vi "final gps synchronization with recursive algorithm.vi"() -> ()   [LabVIEW 2014]
uses:
  <vilib>/FPGAPlugInAG/cRIO-9063/niLvFpga_Open_cRIO-9063.vi
  <vilib>/rvi/interface/common/dynamic/niFpgaDynamicAddResources.vi
  <vilib>/Utility/error.llb/Error Cluster From Error Code.vi
  <vilib>/rvi/errors/niLvFpgaAdjustHostInterfaceError.vi
  <vilib>/FPGAPlugInAG/Dynamic/niLvFpga_Close_Dynamic.vi
  <vilib>/rvi/interface/nirviOpenFPGA/nirviOpenFPGA.xnode
  akhil3/FPGA Bitfiles/trailswithgps_FPGATarget_recursiveakhil_QexfQQGvF84.lvbitx
  recursive akhil.vi
  akhil3/FPGA Bitfiles/trailswithgps_FPGATarget2_recursive2_3NDbUzkOS+M.lvbitx
  recursive2.vi
  <vilib>/rvi/interface/nirviReadWriteControl/nirviReadWriteControl.xnode
  <vilib>/rvi/interface/nirviCloseFPGA/nirviCloseFPGA.xnode
  NiFpgaLv.dll
  <vilib>/rvi/interface/Simulation/niFpgaSimulationCallBeginRW.vi
panel:
  out "Apparent Power":dynamicdata(graph)
  out "LabVIEW time":timestamp
  out "GPS status":T1(ring)
  out "FPGA Timekeeper locked":bool
  out "offset from time reference":i32
  out "Satellites Available":u8
  out "UTC offset":i8
  out "UTC offset valid":bool
  out "Frequency":fxp<+/-,35,18>
  out "current frequency":fxp<+/-,35,18>
  out "PPS Timestamp (TAI ns)":u64
  out "PPS TAI Timestamp":timestamp format="%<%.9X\n%x>T"
  out "PPS UTC Timestamp":timestamp format="%<%.9X\n%x>T"
  out "antenna status":T2(ring)
  out "Latitude (°)":fxp<+/-,28,8>
  out "Longitude (°)":fxp<+/-,29,9>
  out "Altitude (m)":fxp<+/-,24,17>
  out "ROCOF":fxp<+/-,17,17>
  out "Theta":fxp<+/-,22,10>[](array[numeric])
  out "Magnitude":fxp<+,60,17>[](array[numeric])
  out "Current Phasors":picture
  in  "polar attributes 6":T3={"maximum"=0.0, "minimum"=0.0, "clip to min"=FALSE, "log?(F)"=FALSE, "grid color"=6710886, "plot color"=65280, "fmt and prec"={"format"=enum."Decimal", "precision"=0}, "visible section"=8} {"minimum" format="%0.2f"; "maximum" format="%0.2f"}
  out "Voltage Phasors":picture
  in  "polar attributes 7":T3={"maximum"=0.0, "minimum"=0.0, "clip to min"=FALSE, "log?(F)"=FALSE, "grid color"=6710886, "plot color"=65280, "fmt and prec"={"format"=enum."Decimal", "precision"=0}, "visible section"=8} {"minimum" format="%0.2f"; "maximum" format="%0.2f"}
  out "?":cluster{fxp<+/-,22,10>[]}[](array[cluster])
  out "?":cluster{fxp<+,60,17>[]}[](array[cluster])
  out "?":cluster{fxp<+/-,22,10>[]}[](array[cluster])
  out "?":cluster{fxp<+,60,17>[]}[](array[cluster])
  out "Voltages at PMU 1":dynamicdata(graph)
  out "LabVIEW time 2":timestamp
  out "GPS status 2":T1(ring)
  out "FPGA Timekeeper locked 2":bool
  out "offset from time reference 2":i32
  out "Satellites Available 2":u8
  out "UTC offset 2":i8
  out "UTC offset valid 2":bool
  out "Frequency":fxp<+/-,35,18>
  out "current frequency 2":fxp<+/-,35,18>
  out "PPS Timestamp (TAI ns) 2":u64
  out "PPS TAI Timestamp 2":timestamp format="%<%.9X\n%x>T"
  out "PPS UTC Timestamp 2":timestamp format="%<%.9X\n%x>T"
  out "antenna status 2":T2(ring)
  out "Latitude (°) 2":fxp<+/-,28,8>
  out "Longitude (°) 2":fxp<+/-,29,9>
  out "Altitude (m) 2":fxp<+/-,24,17>
  out "ROCOF":fxp<+/-,17,17>
  out "Theta 2":fxp<+/-,22,10>[](array[numeric])
  out "Magnitude 2":fxp<+,60,17>[](array[numeric])
  out "Current Phasors":picture
  in  "polar attributes 8":T3={"maximum"=0.0, "minimum"=0.0, "clip to min"=FALSE, "log?(F)"=FALSE, "grid color"=6710886, "plot color"=65280, "fmt and prec"={"format"=enum."Decimal", "precision"=0}, "visible section"=8} {"minimum" format="%0.2f"; "maximum" format="%0.2f"}
  out "Voltage Phasors":picture
  in  "polar attributes 9":T3={"maximum"=0.0, "minimum"=0.0, "clip to min"=FALSE, "log?(F)"=FALSE, "grid color"=6710886, "plot color"=65280, "fmt and prec"={"format"=enum."Decimal", "precision"=0}, "visible section"=8} {"minimum" format="%0.2f"; "maximum" format="%0.2f"}
  out "?":cluster{fxp<+/-,22,10>[]}[](array[cluster])
  out "?":cluster{fxp<+,60,17>[]}[](array[cluster])
  out "?":cluster{fxp<+/-,22,10>[]}[](array[cluster])
  out "?":cluster{fxp<+,60,17>[]}[](array[cluster])
  out "Voltages at PMU 2":dynamicdata(graph)
  out "Frequency":dynamicdata(graph)
  out "Reactive Power":dbl
  out "Real Power":dbl
  out "Power factor":dbl
  out "Apparent Power":dbl
  out "Reactive Power":dbl
  out "Real Power":dbl
  out "Power factor":dbl
  out "Apparent Power":dbl
  out "Load angle 2":dbl(graph)
  out "Load angle":dbl
  out "x/y":fxp<+/-,48,24>
  out "x/y 2":fxp<+/-,48,24>
  out "x-y":fxp<+/-,49,25>
  out "Waveform Chart 3":dbl(graph)
  out "x/y 3":fxp<+/-,48,24>
  out "x/y 4":fxp<+/-,48,24>
  out "x-y 2":fxp<+/-,49,25>
  out "x-y 3":fxp<+/-,50,26>
  out "Waveform Chart 4":dynamicdata(graph)
  out "Real Power":dynamicdata(graph)
  out "Reactive Power":dynamicdata(graph)
  out "GPS TIMESTAMP":timestamp[](array[timestamp])
  out "Frequency":fxp<+/-,35,18>[](array[numeric])
  out "ROCOF":fxp<+/-,17,17>[](array[numeric])
  out "Frequency 2":fxp<+/-,50,19>[](array[numeric])
  out "ROCOF2":fxp<+/-,26,12>[](array[numeric])
  # "PHASOR DATA CONCENTRATOR (RECURSIVE ALGORITHM)"
  # "PHASOR MEASUREMENT UNIT 1"
  # "PHASOR MEASUREMENT UNIT 2"
  # "GPS SYNCHRONIZATION"
  # "Voltage Phasors"
  # "Voltage Phasors"
  # "R Phase"
  # "R Phase"
  # "Y Phase"
  # "Y Phase"
  # "B Phase"
  # "B Phase"
  # "Frequency and ROCOF"
  # "Frequency and ROCOF"
  # "Current Phasors"
  # "Current Phasors"
  # "PMU 1"
  # "R Phase"
  # "PMU 2"
  # "R Phase"
  # "Y Phase"
  # "Y Phase"
  # "B Phase"
  # "B Phase"
  # "PHASOR DATA CONCENTRATOR (RECURSIVE ALGORITHM)"
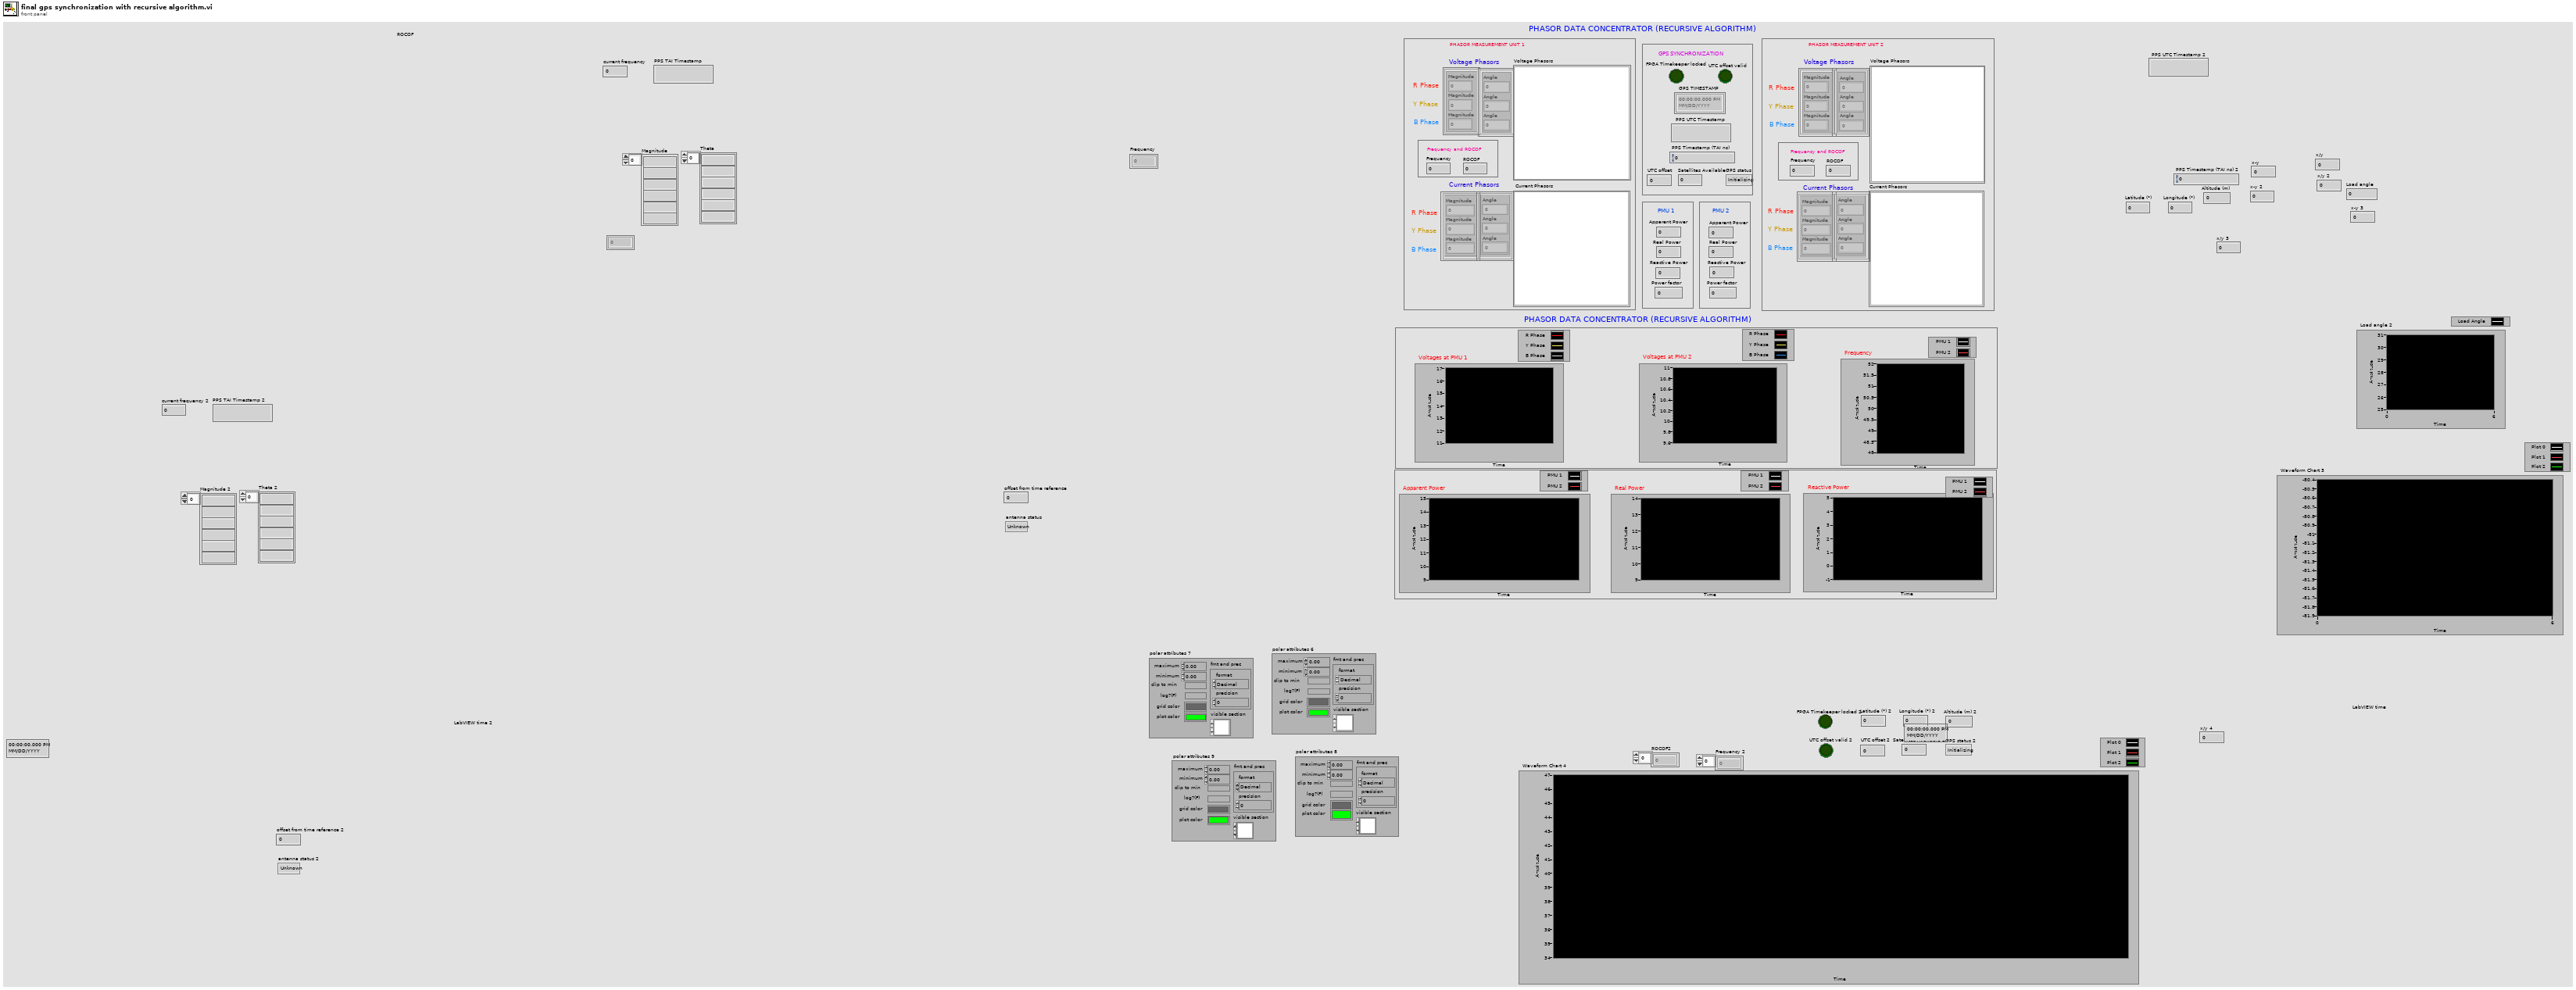
[diagram p1: front panel]
types:
  T1 = enum8{"Initializing", "Normal", "Unable to get fix"}
  T2 = enum8{"Unknown", "Normal", "Absent", "Overcurrent"}
  T3 = cluster{"maximum":dbl, "minimum":dbl, "clip to min":bool, "log?(F)":bool, "grid color":u32, "plot color":u32, "fmt and prec":cluster{"format":enum8{"Decimal", "Scientific", "Engineering", "Binary", "Octal", "Hex"}, "precision":u8}, "visible section":u16}
  T4 = cluster{"magnitude":fxp<+,60,17>, "element":fxp<+/-,61,18>}[]
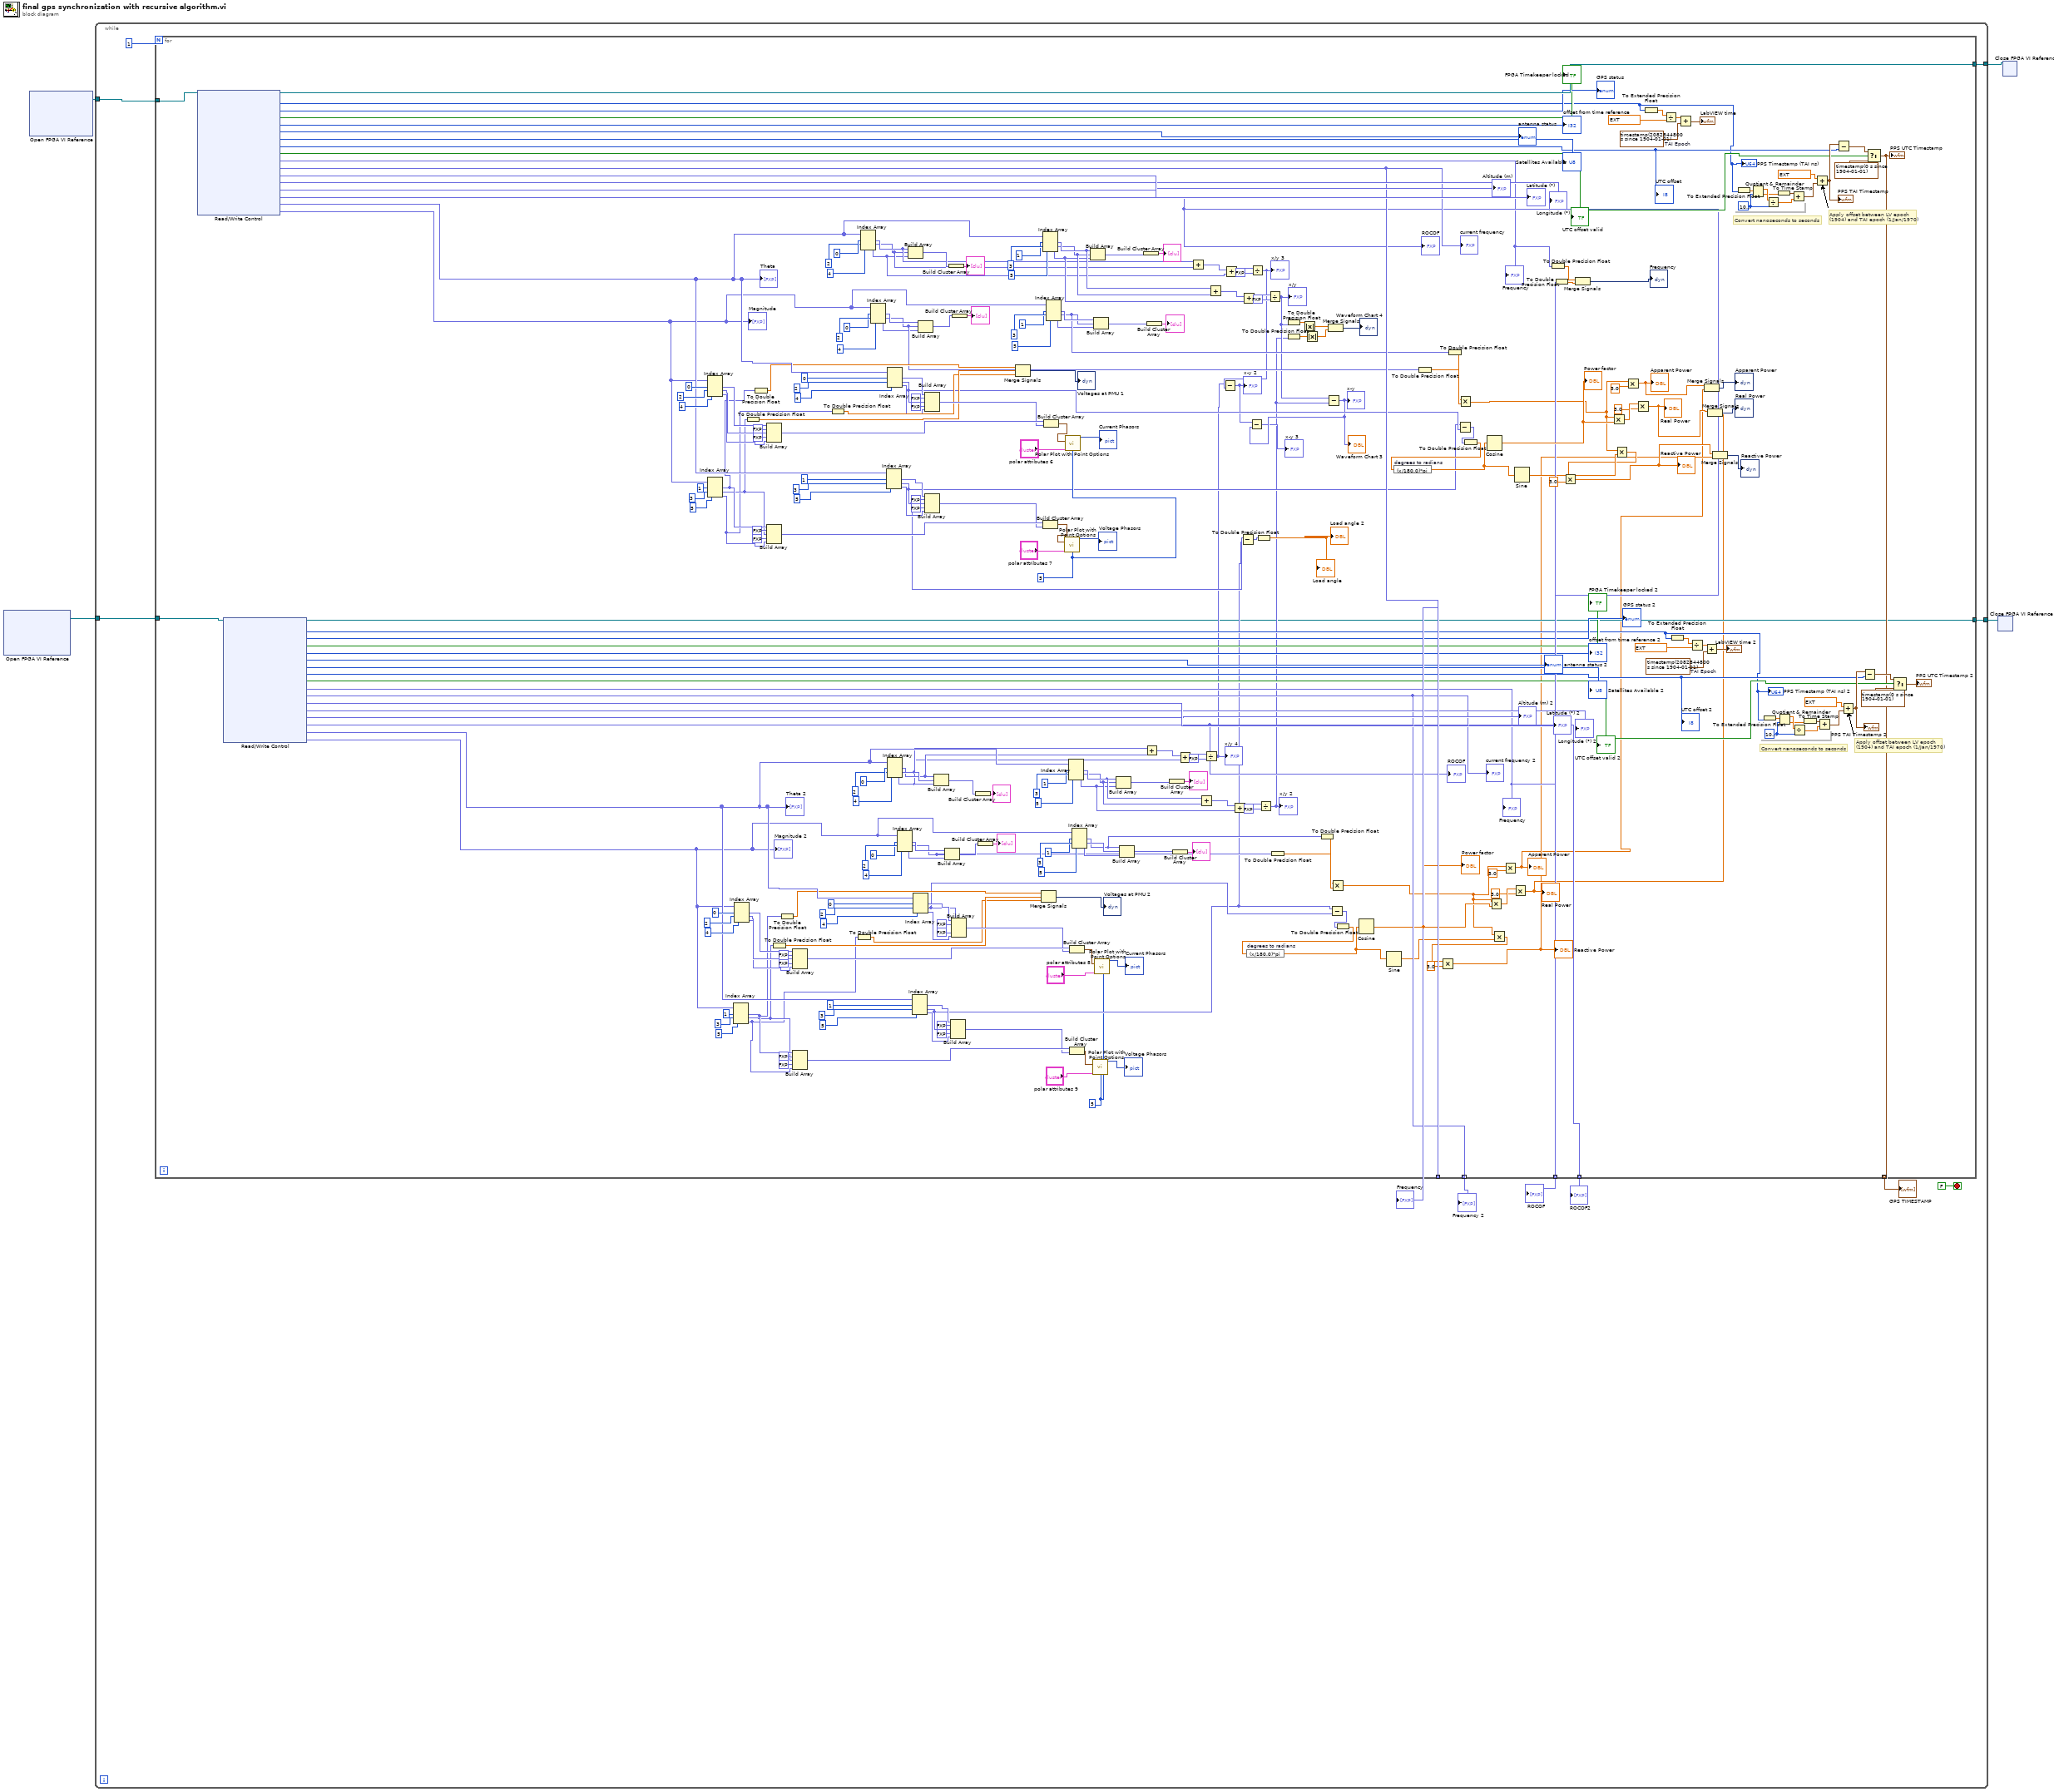
[diagram p0: block diagram]
diagram:
  n1 = xnode "Open FPGA VI Reference"() -> ("FPGA VI Reference Out"=w2:refnum<k20>)  [unwired: 2 in, 1 out]
  n2 = xnode "Open FPGA VI Reference"() -> ("FPGA VI Reference Out"=w3:refnum<k20>)  [unwired: 2 in, 1 out]
  n3 = while {
    tunnel: [w14] -> w4
    tunnel: w3 -> [w12]
    tunnel: w2 -> [w7]
    tunnel: [w5] -> w1
    stop <- FALSE stop-if-true
    n4 = for {
      N: 1 ("Numeric") -> [_]
      tunnel: w12 -> [w302]
      tunnel: [w301] -> w14
      tunnel: [w32] -> w15 mode=indexing
      tunnel: [w225] -> w11 mode=indexing
      tunnel: [w224] -> w10 mode=indexing
      tunnel: w7 -> [w128]
      tunnel: [w127] -> w9 mode=indexing
      tunnel: [w126] -> w8 mode=indexing
      tunnel: [w31] -> w5
      w70 = u16 5 ("Size 2")
      w226 = u16 5 ("Size")
      w205 = u32 1000000000
      w214 = timestamp(2082844800 s since 1904-01-01)  # TAI Epoch
      w294 = u32 1000000000
      w305 = timestamp(2082844800 s since 1904-01-01)  # TAI Epoch
      # "Apply offset between LV epoch (1904) and TAI epoch (1/Jan/1970)"
      # "Convert nanoseconds to seconds"
      # "Apply offset between LV epoch (1904) and TAI epoch (1/Jan/1970)"
      # "Convert nanoseconds to seconds"
      n5 = xnode "Read/Write Control"("FPGA VI Reference In"=w302) -> ("FPGA VI Reference Out"=w301:refnum<k20>, "FPGA Timekeeper time (ns) 2"=w282:u64, "GPS status"=→"GPS status":T1, "FPGA Timekeeper locked"=→"FPGA Timekeeper locked":bool, "offset from time reference"=→"offset from time reference":i32, "antenna status"=→"antenna status":T2, "satellites available"=→"Satellites Available":u8, "UTC offset"=w284:i8, "UTC offset valid"=w285:bool, "Voltage Frequency"=w109:fxp<+/-,35,18>, "current frequency"=w225:fxp<+/-,35,18>, "Latitude (°)"=→"Latitude (°)":fxp<+/-,28,8>, "Longitude (°)"=→"Longitude (°)":fxp<+/-,29,9>, "Altitude (m)"=→"Altitude (m)":fxp<+/-,24,17>, "ROCOF"=w224:fxp<+/-,17,17>, "theta"=w242:fxp<+/-,22,10>[], "r"=w235:fxp<+,60,17>[])  [unwired: 1 in, 1 out]
      "UTC offset" <- w284
      "UTC offset valid" <- w285
      "Frequency" <- w109
      "current frequency" <- w225
      "PPS Timestamp (TAI ns)" <- w282
      "ROCOF" <- w224
      "Theta" <- w242
      "Magnitude" <- w235
      n6 = xnode "Read/Write Control"("FPGA VI Reference In"=w128) -> ("FPGA VI Reference Out"=w31:refnum<k20>, "FPGA Timekeeper time (ns) 2"=w193:u64, "GPS status"=→"GPS status 2":T1, "FPGA Timekeeper locked"=→"FPGA Timekeeper locked 2":bool, "offset from time reference"=→"offset from time reference 2":i32, "antenna status"=→"antenna status 2":T2, "satellites available"=→"Satellites Available 2":u8, "UTC offset"=w195:i8, "UTC offset valid"=w196:bool, "Voltage Frequency"=w108:fxp<+/-,35,18>, "current frequency"=w127:fxp<+/-,35,18>, "Latitude (°)"=→"Latitude (°) 2":fxp<+/-,28,8>, "Longitude (°)"=→"Longitude (°) 2":fxp<+/-,29,9>, "Altitude (m)"=→"Altitude (m) 2":fxp<+/-,24,17>, "ROCOF"=w126:fxp<+/-,17,17>, "theta"=w155:fxp<+/-,22,10>[], "r"=w144:fxp<+,60,17>[])  [unwired: 1 in, 1 out]
      "UTC offset 2" <- w195
      "UTC offset valid 2" <- w196
      "Frequency" <- w108
      "current frequency 2" <- w127
      "PPS Timestamp (TAI ns) 2" <- w193
      "ROCOF" <- w126
      "Theta 2" <- w155
      "Magnitude 2" <- w144
      n7 = Index Array(array=w235, index #1=1 ("index"), index #2=3 ("index"), index #3=5 ("index")) -> (element #1=w21:fxp<+,60,17>, element #2=w20:fxp<+,60,17>, element #3=w19:fxp<+,60,17>)
      n8 = Index Array(array=w235, index #1=0 ("index"), index #2=2 ("index"), index #3=4 ("index")) -> (element #1=w221:fxp<+,60,17>, element #2=w223:fxp<+,60,17>, element #3=w219:fxp<+,60,17>)
      n9 = Index Array(array=w144, index #1=1 ("index"), index #2=3 ("index"), index #3=5 ("index")) -> (element #1=w18:fxp<+,60,17>, element #2=w17:fxp<+,60,17>, element #3=w16:fxp<+,60,17>)
      n10 = Index Array(array=w144, index #1=0 ("index"), index #2=2 ("index"), index #3=4 ("index")) -> (element #1=w133:fxp<+,60,17>, element #2=w135:fxp<+,60,17>, element #3=w131:fxp<+,60,17>)
      n11 = To Double Precision Float(number=w20) -> (double precision float=w222:dbl)
      n12 = To Double Precision Float(number=w21) -> (double precision float=w220:dbl)
      n13 = Build Array(w21, fxp<+,60,17> 0.0 ("element"), w20, fxp<+,60,17> 0.0 ("element"), w19) -> (w253:fxp<+,60,17>[])
      n14 = Build Array(w221, fxp<+,60,17> 0.0 ("element"), w223, fxp<+,60,17> 0.0 ("element"), w219) -> (w268:fxp<+,60,17>[])
      n15 = To Double Precision Float(number=w17) -> (double precision float=w134:dbl)
      n16 = To Double Precision Float(number=w18) -> (double precision float=w132:dbl)
      n17 = Build Array(w18, fxp<+,60,17> 0.0 ("element"), w17, fxp<+,60,17> 0.0 ("element"), w16) -> (w163:fxp<+,60,17>[])
      n18 = Build Array(w133, fxp<+,60,17> 0.0 ("element"), w135, fxp<+,60,17> 0.0 ("element"), w131) -> (w177:fxp<+,60,17>[])
      n19 = To Double Precision Float(number=w19) -> (double precision float=w218:dbl)
      n20 = To Double Precision Float(number=w16) -> (double precision float=w130:dbl)
      n21 = Index Array(array=w242, index #1=0 ("index"), index #2=2 ("index"), index #3=4 ("index")) -> (element #1=w54:fxp<+/-,22,10>, element #2=w53:fxp<+/-,22,10>, element #3=w52:fxp<+/-,22,10>)
      n22 = Index Array(array=w235, index #1=0 ("index"), index #2=2 ("index"), index #3=4 ("index")) -> (element #1=w123:fxp<+,60,17>, element #2=w115:fxp<+,60,17>, element #3=w110:fxp<+,60,17>)
      n23 = Index Array(array=w242, index #1=1 ("index"), index #2=3 ("index"), index #3=5 ("index")) -> (element #1=w125:fxp<+/-,22,10>, element #2=w81:fxp<+/-,22,10>, element #3=w112:fxp<+/-,22,10>)
      n24 = Index Array(array=w242, index #1=0 ("index"), index #2=2 ("index"), index #3=4 ("index")) -> (element #1=w124:fxp<+/-,22,10>, element #2=w116:fxp<+/-,22,10>, element #3=w113:fxp<+/-,22,10>)
      n25 = Index Array(array=w155, index #1=0 ("index"), index #2=2 ("index"), index #3=4 ("index")) -> (element #1=w47:fxp<+/-,22,10>, element #2=w48:fxp<+/-,22,10>, element #3=w46:fxp<+/-,22,10>)
      n26 = Index Array(array=w144, index #1=0 ("index"), index #2=2 ("index"), index #3=4 ("index")) -> (element #1=w148:fxp<+,60,17>, element #2=w91:fxp<+,60,17>, element #3=w149:fxp<+,60,17>)
      n27 = Build Array(w54, w53, w52) -> (w234:fxp<+/-,22,10>[])
      n28 = Index Array(array=w155, index #1=1 ("index"), index #2=3 ("index"), index #3=5 ("index")) -> (element #1=w165:fxp<+/-,22,10>, element #2=w80:fxp<+/-,22,10>, element #3=w164:fxp<+/-,22,10>)
      n29 = Index Array(array=w155, index #1=0 ("index"), index #2=2 ("index"), index #3=4 ("index")) -> (element #1=w179:fxp<+/-,22,10>, element #2=w90:fxp<+/-,22,10>, element #3=w178:fxp<+/-,22,10>)
      n30 = Build Array(w123, w115, w110) -> (w233:fxp<+,60,17>[])
      n31 = Build Array(w125, fxp<+,60,17> 0.0 ("element"), w81, fxp<+,60,17> 0.0 ("element"), w112) -> (w252:fxp<+/-,61,18>[])
      n32 = Build Array(w124, fxp<+,60,17> 0.0 ("element"), w116, fxp<+,60,17> 0.0 ("element"), w113) -> (w267:fxp<+/-,61,18>[])
      n33 = Build Array(w47, w48, w46) -> (w143:fxp<+/-,22,10>[])
      n34 = Build Array(w148, w91, w149) -> (w142:fxp<+,60,17>[])
      n35 = Build Cluster Array(w234) -> (→"?":cluster{fxp<+/-,22,10>[]}[])
      n36 = Build Array(w165, fxp<+,60,17> 0.0 ("element"), w80, fxp<+,60,17> 0.0 ("element"), w164) -> (w162:fxp<+/-,61,18>[])
      n37 = Build Array(w179, fxp<+,60,17> 0.0 ("element"), w90, fxp<+,60,17> 0.0 ("element"), w178) -> (w176:fxp<+/-,61,18>[])
      n38 = Build Cluster Array(w233) -> (→"?":cluster{fxp<+,60,17>[]}[])
      n39 = Build Cluster Array(w143) -> (→"?":cluster{fxp<+/-,22,10>[]}[])
      n40 = Build Cluster Array(w142) -> (→"?":cluster{fxp<+,60,17>[]}[])
      n41 = Merge Signals(w220, w222, w218) -> (→"Voltages at PMU 1":dynamicdata)
      n42 = Merge Signals(w132, w134, w130) -> (→"Voltages at PMU 2":dynamicdata)
      n43 = Index Array(array=w242, index #1=1 ("index"), index #2=3 ("index"), index #3=5 ("index")) -> (element #1=w69:fxp<+/-,22,10>, element #2=w68:fxp<+/-,22,10>, element #3=w66:fxp<+/-,22,10>)
      n44 = Build Cluster Array(w253, w252) -> (w250:T4)
      n45 = Build Cluster Array(w268, w267) -> (w265:T4)
      n46 = Index Array(array=w235, index #1=1 ("index"), index #2=3 ("index"), index #3=5 ("index")) -> (element #1=w122:fxp<+,60,17>, element #2=w114:fxp<+,60,17>, element #3=w111:fxp<+,60,17>)
      n47 = call <vilib>:"Polar Plot with Point Options.vi"("data array [mag, phase (deg)]"=w250, "polar attributes"="polar attributes 7", "Size"=w226) -> ("new picture"=→"Voltage Phasors":picture)  [unwired: 12 in]
      n48 = call <vilib>:"Polar Plot with Point Options.vi"("data array [mag, phase (deg)]"=w265, "polar attributes"="polar attributes 6", "Size"=w226) -> ("new picture"=→"Current Phasors":picture)  [unwired: 12 in]
      n49 = Index Array(array=w155, index #1=1 ("index"), index #2=3 ("index"), index #3=5 ("index")) -> (element #1=w60:fxp<+/-,22,10>, element #2=w59:fxp<+/-,22,10>, element #3=w58:fxp<+/-,22,10>)
      n50 = Build Cluster Array(w163, w162) -> (w76:T4)
      n51 = Build Cluster Array(w177, w176) -> (w73:T4)
      n52 = Index Array(array=w144, index #1=1 ("index"), index #2=3 ("index"), index #3=5 ("index")) -> (element #1=w92:fxp<+,60,17>, element #2=w153:fxp<+,60,17>, element #3=w154:fxp<+,60,17>)
      n53 = Build Array(w69, w68, w66) -> (w230:fxp<+/-,22,10>[])
      n54 = call <vilib>:"Polar Plot with Point Options.vi"("data array [mag, phase (deg)]"=w76, "polar attributes"="polar attributes 9", "Size"=w70) -> ("new picture"=→"Voltage Phasors":picture)  [unwired: 12 in]
      n55 = Build Array(w122, w114, w111) -> (w229:fxp<+,60,17>[])
      n56 = call <vilib>:"Polar Plot with Point Options.vi"("data array [mag, phase (deg)]"=w73, "polar attributes"="polar attributes 8", "Size"=w70) -> ("new picture"=→"Current Phasors":picture)  [unwired: 12 in]
      n57 = Build Array(w60, w59, w58) -> (w139:fxp<+/-,22,10>[])
      n58 = Build Array(w92, w153, w154) -> (w138:fxp<+,60,17>[])
      n59 = Build Cluster Array(w230) -> (→"?":cluster{fxp<+/-,22,10>[]}[])
      n60 = Add(x=w48, y=w47) -> (x+y=w51:fxp<+/-,23,11>)
      n61 = Build Cluster Array(w229) -> (→"?":cluster{fxp<+,60,17>[]}[])
      n62 = Build Cluster Array(w139) -> (→"?":cluster{fxp<+/-,22,10>[]}[])
      n63 = Build Cluster Array(w138) -> (→"?":cluster{fxp<+,60,17>[]}[])
      n64 = Add(x=w51, y=w46) -> (x+y=w50:fxp<+/-,24,12>)
      n65 = Add(x=w54, y=w53) -> (x+y=w57:fxp<+/-,23,11>)
      n66 = Add(x=w60, y=w59) -> (x+y=w63:fxp<+/-,23,11>)
      n67 = Divide(x=w50, y=fxp<+/-,24,12> 3.0) -> (x/y=w44:fxp<+/-,48,24>)
      "x/y 4" <- w44
      n68 = Add(x=w69, y=w68) -> (x+y=w67:fxp<+/-,23,11>)
      n69 = Add(x=w57, y=w52) -> (x+y=w56:fxp<+/-,24,12>)
      n70 = Add(x=w63, y=w58) -> (x+y=w62:fxp<+/-,24,12>)
      n71 = Subtract(x=w81, y=w80) -> (x-y=w79:fxp<+/-,23,11>)
      n72 = Add(x=w67, y=w66) -> (x+y=w65:fxp<+/-,24,12>)
      n73 = Divide(x=w56, y=fxp<+/-,24,12> 3.0) -> (x/y=w45:fxp<+/-,48,24>)
      "x/y 3" <- w45
      n74 = Subtract(x=w44, y=w45) -> (x-y=w43:fxp<+/-,49,25>)
      "x-y 2" <- w43
      n75 = To Double Precision Float(number=w79) -> (double precision float=→"Load angle 2" →"Load angle":dbl)
      n76 = Divide(x=w62, y=fxp<+/-,24,12> 3.0) -> (x/y=w39:fxp<+/-,48,24>)
      "x/y 2" <- w39
      n77 = Divide(x=w65, y=fxp<+/-,24,12> 3.0) -> (x/y=w40:fxp<+/-,48,24>)
      "x/y" <- w40
      n78 = To Double Precision Float(number=w91) -> (double precision float=w95:dbl)
      n79 = To Double Precision Float(number=w40) -> (double precision float=w38:dbl)
      n80 = To Double Precision Float(number=w39) -> (double precision float=w37:dbl)
      n81 = Absolute Value(x=w38) -> (abs(x)=w35:dbl)
      n82 = Absolute Value(x=w37) -> (abs(x)=w34:dbl)
      n83 = To Double Precision Float(number=w92) -> (double precision float=w96:dbl)
      n84 = Subtract(x=w40, y=w39) -> (x-y=w42:fxp<+/-,49,25>)
      "x-y" <- w42
      "Waveform Chart 3" <- w42
      n85 = Subtract(x=w43, y=w42) -> (x-y=→"x-y 3":fxp<+/-,50,26>)
      n86 = Merge Signals(w35, w34) -> (→"Waveform Chart 4":dynamicdata)
      n87 = Subtract(x=w80, y=w90) -> (x-y=w97:fxp<+/-,23,11>)
      n88 = Multiply(x=w95, y=w96) -> (x*y=w82:dbl)
      n89 = To Double Precision Float(number=w97) -> (double precision float=w93:dbl)
      n90 = expression code="(x/180.0)*pi" "degrees to radians"(w93) -> (w94:dbl)
      n91 = Cosine(x=w94) -> (cos(x)=w83:dbl)
      "Power factor" <- w83
      n92 = Sine(x=w94) -> (sin(x)=w85:dbl)
      n93 = To Double Precision Float(number=w115) -> (double precision float=w118:dbl)
      n94 = To Double Precision Float(number=w114) -> (double precision float=w119:dbl)
      n95 = Subtract(x=w81, y=w116) -> (x-y=w121:fxp<+/-,23,11>)
      n96 = Multiply(x=w118, y=w119) -> (x*y=w99:dbl)
      n97 = To Double Precision Float(number=w121) -> (double precision float=w117:dbl)
      n98 = expression code="(x/180.0)*pi" "degrees to radians"(w117) -> (w105:dbl)
      n99 = Cosine(x=w105) -> (cos(x)=w120:dbl)
      "Power factor" <- w120
      n100 = Multiply(x=w82, y=w83) -> (x*y=w89:dbl)
      n101 = Multiply(x=w82, y=w85) -> (x*y=w84:dbl)
      n102 = Multiply(x=w84, y=3.0) -> (x*y=w27:dbl)
      "Reactive Power" <- w27
      n103 = Multiply(x=w82, y=3.0) -> (x*y=w23:dbl)
      "Apparent Power" <- w23
      n104 = Multiply(x=w89, y=3.0) -> (x*y=w29:dbl)
      "Real Power" <- w29
      n105 = Sine(x=w105) -> (sin(x)=w104:dbl)
      n106 = To Double Precision Float(number=w109) -> (double precision float=w78:dbl)
      n107 = To Double Precision Float(number=w108) -> (double precision float=w107:dbl)
      n108 = Merge Signals(w78, w107) -> (→"Frequency":dynamicdata)
      n109 = Multiply(x=w99, y=w120) -> (x*y=w101:dbl)
      n110 = Multiply(x=w99, y=w104) -> (x*y=w103:dbl)
      n111 = Multiply(x=w103, y=3.0) -> (x*y=w28:dbl)
      "Reactive Power" <- w28
      n112 = Multiply(x=w99, y=3.0) -> (x*y=w24:dbl)
      "Apparent Power" <- w24
      n113 = Multiply(x=w101, y=3.0) -> (x*y=w30:dbl)
      "Real Power" <- w30
      n114 = To Extended Precision Float(1:w282) -> (0:w303:ext)
      n115 = Divide(x=w303, y=ext 1000000000.0) -> (x/y=w306:ext)
      n116 = To Extended Precision Float(1:w193) -> (0:w212:ext)
      n117 = Add(x=w306, y=w305) -> (x+y=→"LabVIEW time":timestamp)
      n118 = Divide(x=w212, y=ext 1000000000.0) -> (x/y=w215:ext)
      n119 = Merge Signals(w24, w23) -> (→"Apparent Power":dynamicdata)
      n120 = Add(x=w215, y=w214) -> (x+y=→"LabVIEW time 2":timestamp)
      n121 = Merge Signals(w30, w29) -> (→"Real Power":dynamicdata)
      n122 = Merge Signals(w28, w27) -> (→"Reactive Power":dynamicdata)
      n123 = To Extended Precision Float(1:w282) -> (0:w296:ext)
      n124 = Quotient & Remainder(x=w296, y=w294) -> (x-y*floor(x/y)=w295:ext, floor(x/y)=w293:ext)
      n125 = To Extended Precision Float(1:w193) -> (0:w207:ext)
      n126 = Divide(x=w295, y=w294) -> (x/y=w291:ext)
      n127 = To Time Stamp(1:w293) -> (0:w292:timestamp)
      n128 = Quotient & Remainder(x=w207, y=w205) -> (x-y*floor(x/y)=w206:ext, floor(x/y)=w204:ext)
      n129 = Add(x=w292, y=w291) -> (x+y=w290:timestamp)
      n130 = Divide(x=w206, y=w205) -> (x/y=w202:ext)
      n131 = To Time Stamp(1:w204) -> (0:w203:timestamp)
      n132 = Add(x=ext 2082844800.0, y=w290) -> (x+y=w288:timestamp)
      "PPS TAI Timestamp" <- w288
      n133 = Add(x=w203, y=w202) -> (x+y=w201:timestamp)
      n134 = Subtract(x=w288, y=w284) -> (x-y=w287:timestamp)
      n135 = Add(x=ext 2082844800.0, y=w201) -> (x+y=w199:timestamp)
      "PPS TAI Timestamp 2" <- w199
      n136 = Subtract(x=w199, y=w195) -> (x-y=w198:timestamp)
      n137 = Select(t=w287, s=w285, f=timestamp(0 s since 1904-01-01)) -> (s? t:f=w32:timestamp)
      "PPS UTC Timestamp" <- w32
      n138 = Select(t=w198, s=w196, f=timestamp(0 s since 1904-01-01)) -> (s? t:f=→"PPS UTC Timestamp 2":timestamp)
    }
    "GPS TIMESTAMP" <- w15
    "Frequency" <- w11
    "ROCOF" <- w10
    "Frequency 2" <- w9
    "ROCOF2" <- w8
  }
  n139 = xnode "Close FPGA VI Reference"("FPGA VI Reference In"=w1) -> ()  [unwired: 1 in, 1 out]
  n140 = xnode "Close FPGA VI Reference"("FPGA VI Reference In"=w4) -> ()  [unwired: 1 in, 1 out]
